vi "List of Font Families.vi"() -> (3 "Available Fonts":string[](array[string]))   [LabVIEW 2009]
uses:
  C:/Projets/LAVAG/OpenOfficeRGT/AODL/DLLs/AODL.dll
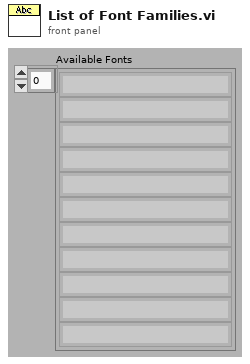
[diagram p1: front panel]
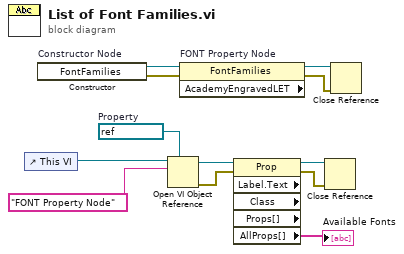
[diagram p0: block diagram]
diagram:
  w10 = refnum<vi> refnum  # Property
  n1 = control-ref of="This VI"() -> (w11:refnum<vi>)
  n2 = constructor on="Constructor Node" class="FontFamilies"() -> (reference out=w12:refnum<k24>, error out=w1:errorcluster)  [unwired: 3 in, 1 out]
  n3 = Open VI Object Reference(7:w10, 10:"FONT Property Node" ("name/order"), 11:w11) -> (0:w4:errorcluster, 3:w8:refnum<vi>)  [unwired: 1 in]
  n4 = property on="FONT Property Node" class="FontFamilies" props=["AcademyEngravedLET"](reference=w12, error in=w1) -> (reference out=w3:refnum<k24>, error out=w2:errorcluster)  [unwired: 1 out]
  n5 = property class="Prop" props=["Label", "Text", "Class", "Props[]", "AllProps[]"](reference=w8, error in=w4) -> (reference out=w6:refnum<vi>, error out=w5:errorcluster, "AllProps[]"=→"Available Fonts":string[])  [unwired: 3 out]
  n6 = Close Reference(reference=w6, error in (no error)=w5) -> ()  [unwired: 1 out]
  n7 = Close Reference(reference=w3, error in (no error)=w2) -> ()  [unwired: 1 out]
